vi "FGV_EventToHmiScheduler.vi"(7 "Command":T1, 8 "error in (no error)":errorcluster) -> (0 "error out":errorcluster, 3 "ToHmiSchedulerEvent":refnum<user-event>)   [LabVIEW 2013]
uses:
  EnumFgvEventCommand.ctl
  ToHmiScheduler.ctl
  ToHmiSchedulerCommand.ctl
  03 - ToMessageHandlerProcess/ToMessageHandlerEvent.ctl
  03 - ToMessageHandlerProcess/enumMessageCriticity.ctl
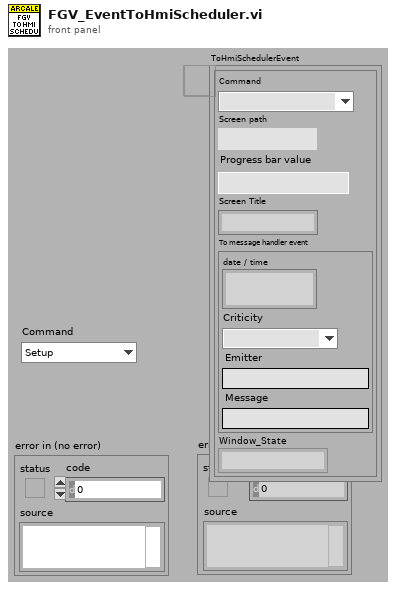
[diagram p1: front panel]
types:
  T1 = typedef "EnumFgvEventCommand.ctl" = enum16{"Setup", "Cleanup", "Get"}
  T2 = typedef "ToHmiScheduler.ctl" = cluster{"Command":T3, "Screen path":path, "Progress bar value":u8, "Screen Title":string, "To message handler event":T4, "Window_State":enum32{"Invalid", "Standard", "Closed", "Hidden", "Minimized", "Maximized"}}
  T3 = typedef "ToHmiSchedulerCommand.ctl" = enum16{"Load screen", "Lock screen", "Unlock screen", "Close enable", "Close disable", "Start automatic progress bar", "Stop automatic progress bar", "Set progress bar value (0..100)", "Load previous screen", "Close application", "View message", "Clear message", "Set Window State"}
  T4 = typedef "ToMessageHandlerEvent.ctl" = cluster{"date / time":timestamp, "Criticity":T5, "Emitter":string, "Message":string}
  T5 = typedef "enumMessageCriticity.ctl" = enum16{"No error", "Info", "Warning", "Error", "Fatal error"}
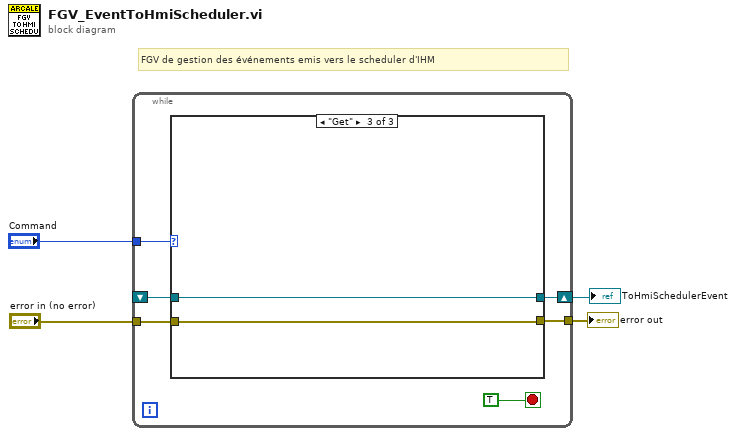
[diagram p0: block diagram]
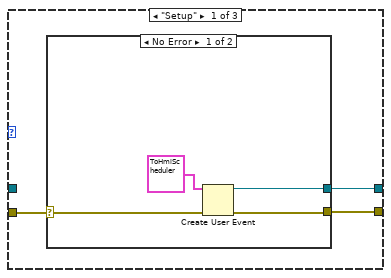
[diagram p2: hidden frame]
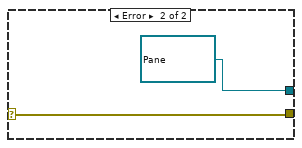
[diagram p3: hidden frame]
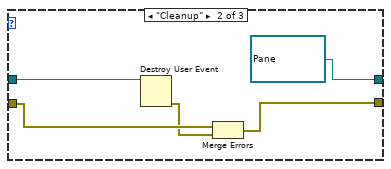
[diagram p4: hidden frame]
diagram:
  # "FGV de gestion des événements emis vers le scheduler d'IHM"
  n1 = while {
    tunnel: "error in (no error)" -> [w8]
    tunnel: "Command" -> [w9]
    tunnel: [w7] -> w2
    shift-right: [w6] -> w1
    shift-left: _ -> [w5]
    stop <- TRUE stop-if-true
    n2 = case shown="\"Get\"" w9 {
      tunnel: w8 -> [w13 w22 w25]
      tunnel: [w12 w20 w25] -> w7
      tunnel: [w11 refnum<user-event> refnum ("ToHmiScheduler") w26] -> w6
      tunnel: w5 -> [_ w24 w26]
      frame "Setup" {
        n3 = case shown="No Error" w13 {
          selector: w13 -> [w17 w19]
          tunnel: [w15 w19] -> w12
          tunnel: [w14 refnum<user-event> refnum ("ToHmiScheduler")] -> w11
          frame No Error {
            n4 = Create User Event(user event datatype=T2 {"Command"=enum."Load screen", "Screen path"=path "", "Progress bar value"=0, "Screen Title"="", "To message handler event"={"date / time"=timestamp(0 s since 1904-01-01), "Criticity"=enum."No error", "Emitter"="", "Message"=""}, "Window_State"=enum."Invalid"} ("ToHmiScheduler"), error in=w17) -> (user event=w14:refnum<user-event>, error out=w15:errorcluster)
          }
          frame Error {
          }
        }
      }
      frame "Cleanup" {
        n5 = Destroy User Event(user event=w24) -> (error out=w21:errorcluster)  [unwired: 1 in]
        n6 = Merge Errors(w22, w21) -> (w20:errorcluster)
      }
      frame "Get" {
      }
    }
  }
  "error out" <- w2
  "ToHmiSchedulerEvent" <- w1
